vi "TogglePump.vi"(7 "LabVIEW Web Service Request":refnum<class "Web Request.lvclass">, 11 "Pump":u8) -> ()   [LabVIEW 2016]
uses:
  <vilib>/wsapi/Web Request.lvclass
  Controller/Messages/Update Vacuum Pump State MSG/Update Vacuum Pump State MSG.lvclass
  G:/sw_repo/For Builds/Nicholas/Controller/Messages/Generic Boolean MSG/Generic Boolean Message.lvclass
  C:/Program Files (x86)/National Instruments/LabVIEW 2016/vi.lib/ActorFramework/Message/Message.lvclass
  Controller/Messages/Generic Boolean MSG/Generic Boolean Message.lvclass/Generic Boolean Message.ctl
  <vilib>/ActorFramework/Message Enqueuer/Message Enqueuer.lvclass/Message Enqueuer.ctl
  Controller/Messages/Generic Boolean MSG/Write Bool.vi
  <vilib>/ActorFramework/Message Priority Queue/Priority Enqueue.vi
  Controller/gController.lvclass
  <vilib>/ActorFramework/Message Enqueuer/Message Enqueuer.lvclass
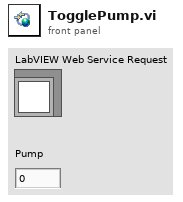
[diagram p1: front panel]
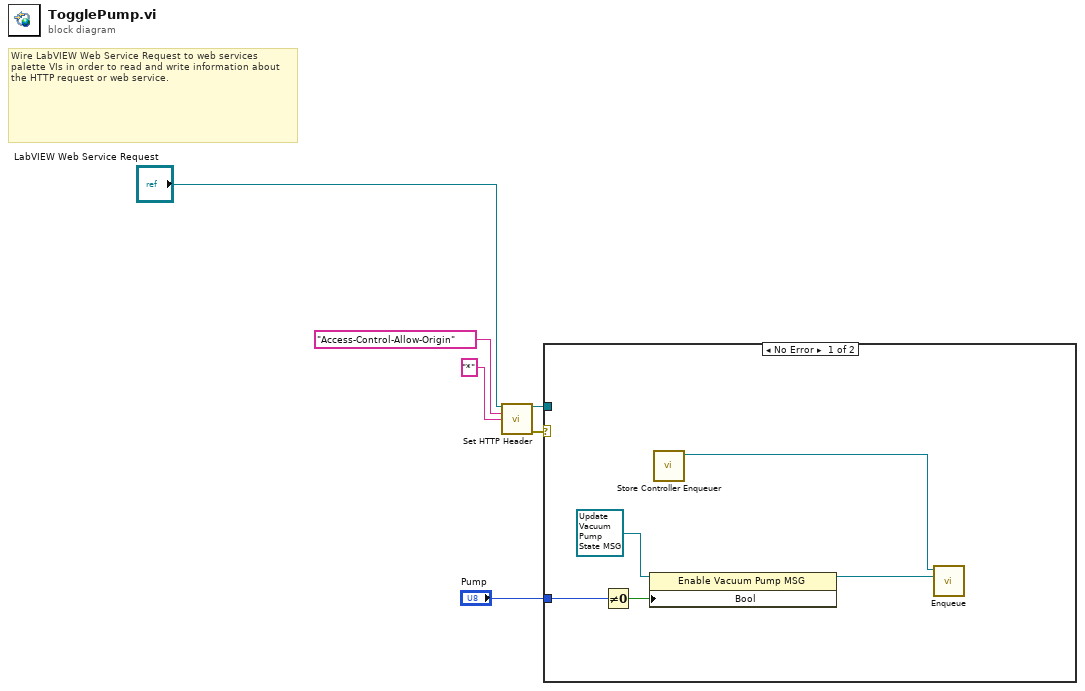
[diagram p0: block diagram]
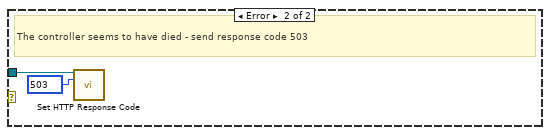
[diagram p2: hidden frame]
diagram:
  # "Wire LabVIEW Web Service Request to web services palette VIs in order to read and write information about the HTTP request or web service."
  n1 = call <vilib>:"Set HTTP Header.vi"("LabVIEW Web Service Request"="LabVIEW Web Service Request", "header"="Access-Control-Allow-Origin", "header value"="*") -> ("LabVIEW Web Service Request out"=w4:refnum<class "Web Request.lvclass">, "error out"=w3:errorcluster)  [unwired: 11 in]
  n2 = case shown="No Error" w3 {
    tunnel: w4 -> [_ w12]
    tunnel: "Pump" -> [w9 _]
    frame No Error {
      n3 = Not Equal To 0?(x=w9) -> (x != 0?=w11:bool)
      n4 = property class="Enable Vacuum Pump MSG"(reference=refnum<class "Update Vacuum Pump State MSG.lvclass"> refnum ("Controller.lvlib:Enable Vacuum Pump MSG"), "Bool"=w11) -> (reference out=w10:refnum<class "Update Vacuum Pump State MSG.lvclass">)  [unwired: 1 in, 1 out]
      n5 = call "Store Controller Enqueuer.vi"() -> ("Controller Enqueuer Out"=w8:refnum<class "Message Enqueuer.lvclass">)  [unwired: 11 in]
      n6 = call <vilib>:"Enqueue.vi"("Message"=w10, "Message Enqueuer in"=w8) -> ()  [unwired: 8 in, 2 out]
    }
    frame Error {
      w13 = 503 items=["100"=100, "101"=101, "200"=200, "201"=201, "202"=202, "203"=203, "204"=204, "205"=205, "206"=206, "300"=300, "301"=301, "302"=302, "303"=303, "304"=304, "305"=305, "306"=306, "307"=307, "400"=400, "401"=401, "402"=402, "403"=403, "404"=404, "405"=405, "406"=406, "407"=407, "408"=408, "409"=409, "410"=410, "411"=411, "412"=412, "413"=413, "414"=414, "415"=415, "416"=416, "417"=417, "500"=500, "501"=501, "502"=502, "503"=503, "504"=504, "505"=505] ("response code (200)")
      # "The controller seems to have died - send response code 503"
      n7 = call <vilib>:"Set HTTP Response Code.vi"("LabVIEW Web Service Request"=w12, "response code (200)"=w13) -> ()  [unwired: 12 in, 2 out]
    }
  }
